vi "ERA_Sys_Order.vi"(7 "Threshold":i32, 8 "Error In":errorcluster, 10 "Vector S":dbl[](array[numeric])) -> (0 "Error Out":errorcluster, 2 "System Order":i32)   [LabVIEW 2017, in "AppPlugins.lvlib" / "EraPlugin.lvclass"]
uses:
  EraPlugin.lvclass
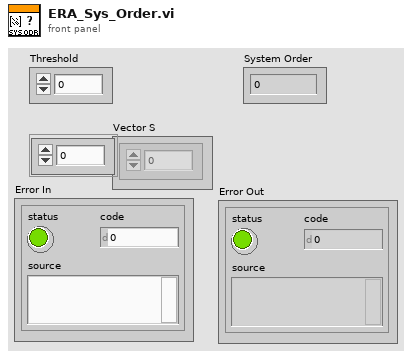
[diagram p1: front panel]
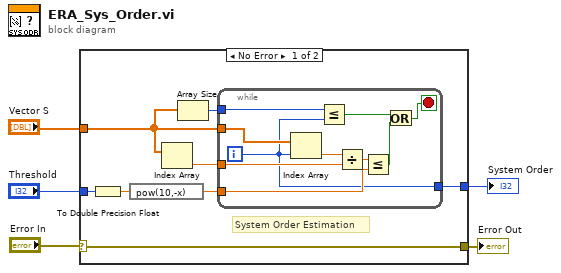
[diagram p0: block diagram]
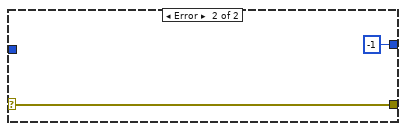
[diagram p2: hidden frame]
diagram:
  n1 = case shown="No Error" "Error In" {
    selector: "Error In" -> [w6 w25]
    tunnel: [w13 -1] -> w5
    tunnel: "Threshold" -> [w11 _]
    tunnel: "Vector S" -> [w7 _]
    tunnel: [w6 w25] -> w1
    frame No Error {
      # "System Order Estimation"
      n2 = To Double Precision Float(number=w11) -> (double precision float=w12:dbl)
      n3 = expression code="pow(10,-x)"(w12) -> (w10:dbl)
      n4 = Index Array(array=w7) -> (element=w9:dbl)  [unwired: 1 in]
      n5 = Array Size(array=w7) -> (size(s)=w8:i32)
      n6 = while {
        tunnel: w9 -> [w20]
        tunnel: w7 -> [w22]
        tunnel: w10 -> [w18]
        tunnel: [w15] -> w13
        tunnel: w8 -> [w14]
        i -> [w15]
        stop <- w16 stop-if-true
        n7 = Index Array(array=w22, index=w15) -> (element=w21:dbl)
        n8 = Less Or Equal?(x=w14, y=w15) -> (x <= y?=w23:bool)
        n9 = Divide(x=w21, y=w20) -> (x/y=w19:dbl)
        n10 = Less Or Equal?(x=w19, y=w18) -> (x <= y?=w17:bool)
        n11 = Or(x=w23, y=w17) -> (x .or. y?=w16:bool)
      }
    }
    frame Error {
    }
  }
  "System Order" <- w5
  "Error Out" <- w1
